vi "Set Tree Item Name.vi"(8 "error in (no error)":errorcluster, 9 "Item Name":string, 10 "Tag":string, 11 "TreeControl in":refnum<vi>) -> (0 "error out":errorcluster, 2 "Tag out":string, 3 "TreeControl out":refnum<vi>)   [LabVIEW 2018]
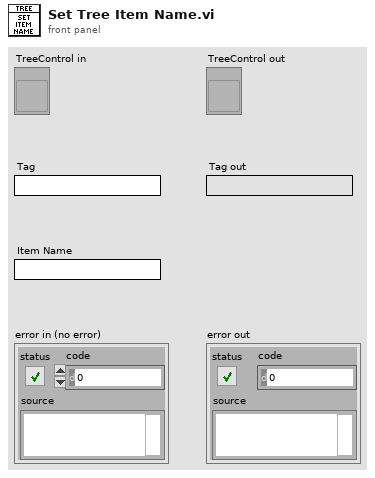
[diagram p1: front panel]
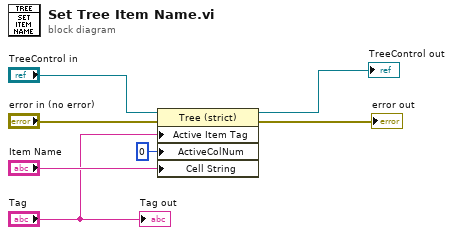
[diagram p0: block diagram]
diagram:
  n1 = property class="Tree (strict)"(reference="TreeControl in", error in="error in (no error)", "Active Item Tag"="Tag", "ActiveColNum"=0 ("Active Cell:Active Column Number"), "Cell String"="Item Name") -> (reference out=→"TreeControl out":refnum<vi>, error out=→"error out":errorcluster)
  "Tag out" <- "Tag"
